vi "Clear_Info.vi"(8 "error in (no error)":errorcluster, 9 "index in":string, 10 "buildObject":T1) -> (0 "error out":errorcluster, 1 "index out":string, 2 "buildObject out":T1)   [LabVIEW 2020, in "IB_DistPart.lvclass"]
uses:
  <vilib>/AppBuilder/IB_Classes/DistPart/IB_DistPart.lvclass
  <vilib>/AppBuilder/IB_Classes/DistPart/IB_DistPart.lvclass/IB_DistPart.ctl
  <vilib>/AppBuilder/IB_RW_Project/IB_RW_Project_PropBag_Action.ctl
  <resource>/Framework/Providers/API/ItemRef.ctl
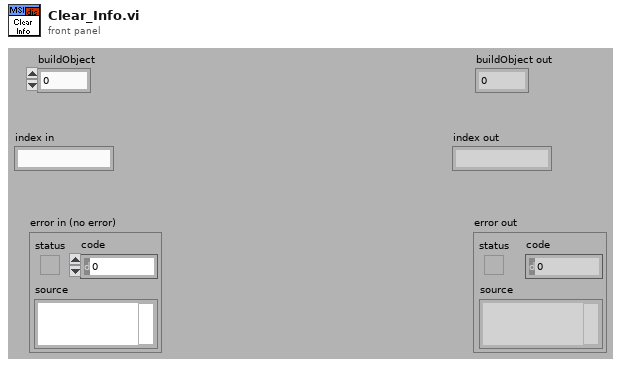
[diagram p1: front panel]
types:
  T1 = typedef "ItemRef.ctl" = u64
  T2 = typedef "IB_RW_Project_PropBag_Action.ctl" = enum16{"read", "write", "clear", "readPrevious", "writePrevious", "clearPrevious"}
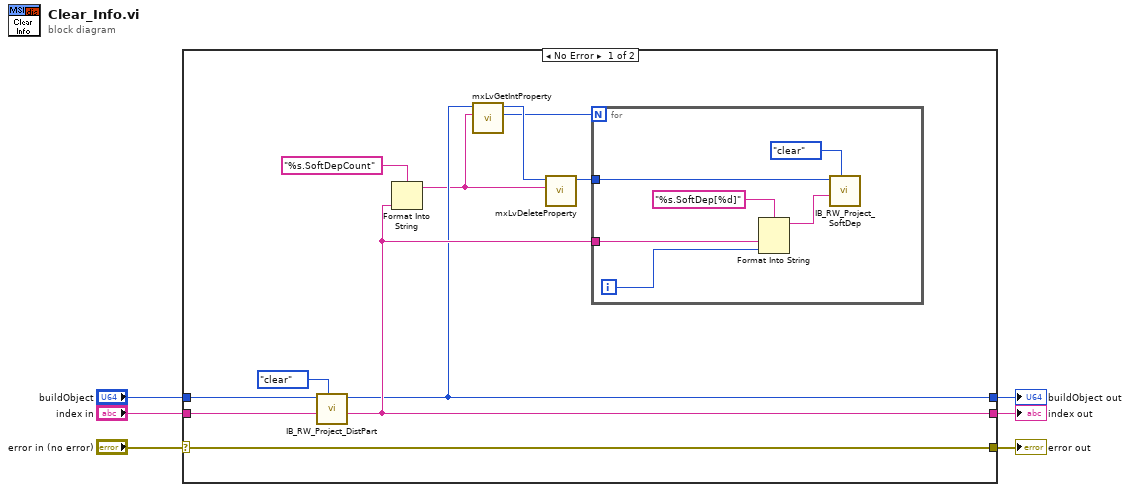
[diagram p0: block diagram]
diagram:
  n1 = case shown="No Error" "error in (no error)" {
    selector: "error in (no error)" -> [w14 w26]
    tunnel: [w14 w26] -> w5
    tunnel: "buildObject" -> [w16 w24]
    tunnel: [w10 w24] -> w3
    tunnel: [w11 w25] -> w2
    tunnel: "index in" -> [w15 w25]
    frame No Error {
      n2 = call <vilib>:"IB_RW_Project_DistPart.vi"("action"=IB_RW_Project_PropBag_Action."clear", "index in"=w15, "buildObject"=w16) -> ("index out"=w11:string, "buildObject out"=w10:T1)  [unwired: 2 in, 5 out]
      n3 = Format Into String(format string="%s.SoftDepCount", w11) -> (resulting string=w8:string)  [unwired: 2 in, 1 out]
      n4 = call <resource>:"mxLvGetIntProperty.vi"("Tag"=w8, "Item"=w10) -> ("Value"=w7:i32, "Item"=w9:T1)  [unwired: 1 in, 7 out]
      n5 = call <resource>:"mxLvDeleteProperty.vi"("Tag"=w8, "Item"=w9) -> ("Item"=w12:T1)  [unwired: 1 in, 8 out]
      n6 = for {
        N: w7 -> [_]
        tunnel: w12 -> [w19]
        tunnel: w11 -> [w18]
        i -> [w21]
        n7 = Format Into String(format string="%s.SoftDep[%d]", w18, w21) -> (resulting string=w20:string)  [unwired: 2 in, 1 out]
        n8 = call <vilib>:"IB_RW_Project_SoftDep.vi"("action"=IB_RW_Project_PropBag_Action."clear", "index in"=w20, "buildObject"=w19) -> ()  [unwired: 2 in, 7 out]
      }
    }
    frame Error {
    }
  }
  "error out" <- w5
  "index out" <- w2
  "buildObject out" <- w3
